vi "MathematicaHandlerNodeTest.vi"() -> ()   [LabVIEW 2014]
uses:
  <vilib>/event_ctls.llb/lveventtype.ctl
panel:
  out "Array":string[](array[string])
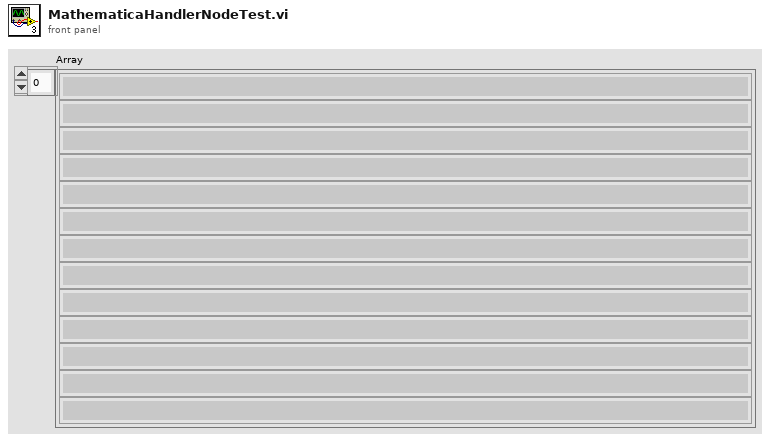
[diagram p1: front panel]
types:
  T1 = typedef "lveventtype.ctl" = enum32{"Null", "Timeout", "Annotation Menu Selection", "Annotation Menu Selection?", "App Instance Close", "App Instance Close?", "Autoscale Range Change", "Bookmark Info Change", "Cell Edit", "Cell Edit?", "Cursor Grab", "Cursor Grab?", "Cursor Menu Selection", "Cursor Menu Selection?", "Cursor Move", "Cursor Release", "Data Change", "Direction Change", "Display State Change", "Drag Ended", "Drag Enter", "Drag Leave", "Drag Over", "Drag Source Update", "Drag Starting", "Drag Starting?", "Drop", "Exec State Change", "Key Down", "Key Down?", "Key Repeat", "Key Repeat?", "Key Up", "Listbox Double Click", "Menu Activation?", "Menu Selection (App)", "Menu Selection? (App)", "Menu Selection (User)", "Mouse Down", "Mouse Down?", "Mouse Enter", "Mouse Leave", "Mouse Move", "Mouse Up", "Mouse Wheel", "NI Security User Change (App)", "Pane Size", "Panel Close", "Panel Close?", "Panel Resize", "Plot Attribute Change", "Scale Range Change", "Shortcut Menu Activation?", "Shortcut Menu Selection (App)", "Shortcut Menu Selection? (App)", "Shortcut Menu Selection (User)", "Tree Double Click", "Tree Drag", "Tree Drag?", "Tree Drop", "Tree Drop?", "Tree Item Close", "Tree Item Close?", "Tree Item Open", "Tree Item Open?", "User Event", "Value Change"}
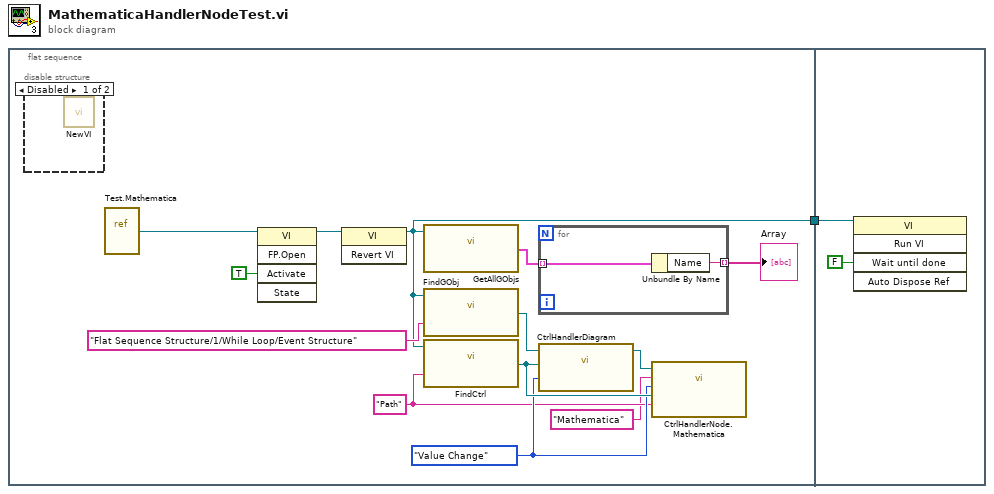
[diagram p0: block diagram]
diagram:
  n1 = flat-sequence {
    tunnel: [w2] -> w1
    tunnel: w1 -> [w17]
    frame #0 {
      w8 = lveventtype."Value Change" ("Type")
      w7 = "Path" ("Name")
      n2 = disable-structure shown="Disabled" {
        frame Disabled {
          n3 = call "NewVI.vi"() -> ()  [unwired: 3 in, 1 out]
        }
        frame Enabled {
        }
      }
      n4 = vi-ref "Test.Mathematica.vi"() -> (w3:refnum<vi>)
      n5 = invoke class="VI" method="FP.Open"(reference=w3, "Activate"=TRUE ("Activate?")) -> (reference out=w4:refnum<vi>)  [unwired: 3 in, 4 out]
      n6 = invoke class="VI" method="Revert VI"(reference=w4) -> (reference out=w2:refnum<vi>)  [unwired: 2 in, 2 out]
      n7 = call "GetAllGObjs.vi"("VI"=w2) -> ("GObjs"=w14:cluster{"Name":string, "GObj":refnum<vi>}[])  [unwired: 1 in]
      n8 = call "FindGObj.vi"("Name"="Flat Sequence Structure/1/While Loop/Event Structure", "VI"=w2) -> ("GObj"=w11:refnum<vi>)
      n9 = call "FindCtrl.vi"("Name"=w7, "VI"=w2) -> ("Ctrl"=w9:refnum<vi>)
      n10 = for {
        tunnel: w14 -> [w16] mode=indexing
        tunnel: [w15] -> w13 mode=indexing
        n11 = Unbundle By Name(w16) -> ("Name"=w15:string)
      }
      "Array" <- w13
      n12 = call "CtrlHandlerDiagram.vi"("Type"=w8, "Ctrl"=w9, "Structure"=w11) -> ("Diagram"=w10:refnum<vi>)  [unwired: 1 out]
      n13 = call "CtrlHandlerNode.Mathematica.vi"("Diagram"=w10, "Name"=w7, "Ctrl"=w9, "Type"=w8, "Data"="Mathematica" ("Name")) -> ()
    }
    frame #1 {
      n14 = invoke class="VI" method="Run VI"(reference=w17, "Wait until done"=FALSE ("Wait Until Done")) -> ()  [unwired: 3 in, 5 out]
    }
  }
